vi "setIdx.vi"() -> ()   [LabVIEW 2016]
uses:
  OptStateEsti/OptStateEsti.lvclass
panel:
  out "dofIdx":i16[](array[numeric])
  out "DOF in Groups 2":T1
  out "zn3Idx 2":bool[](array[boolean])
  in  "DOF in Groups":T1
  in  "zn3Idx":bool[](array[boolean])
  in  "OptStateEsti in":refnum<class "OptStateEsti.lvclass">
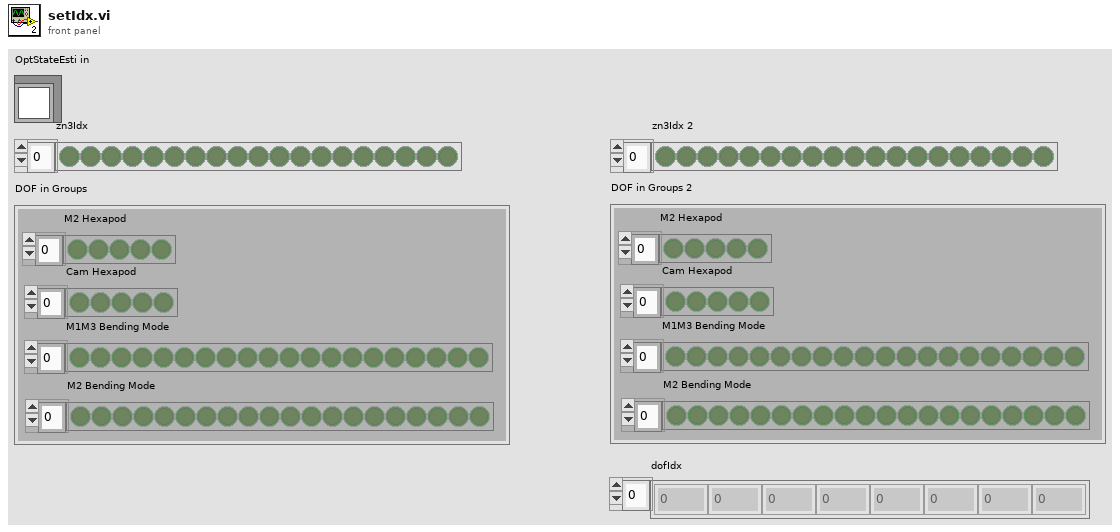
[diagram p1: front panel]
types:
  T1 = cluster{"M2 Hexapod":bool[], "Cam Hexapod ":bool[], "M1M3 Bending Mode":bool[], "M2 Bending Mode":bool[]}
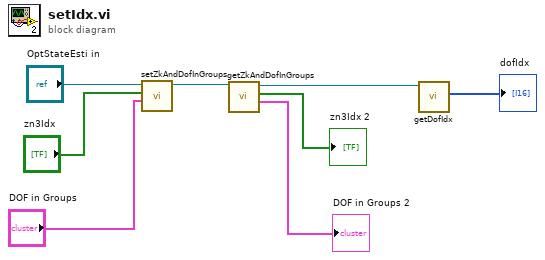
[diagram p0: block diagram]
diagram:
  n1 = call "setZkAndDofInGroups.vi"("DOF in Groups"="DOF in Groups", "zn3Idx"="zn3Idx", "OptStateEsti in"="OptStateEsti in") -> ("OptStateEsti out"=w8:refnum<class "OptStateEsti.lvclass">)  [unwired: 7 in, 1 out]
  n2 = call "getZkAndDofInGroups.vi"("OptStateEsti in"=w8) -> ("DOF in Groups"=→"DOF in Groups 2":T1, "zn3Idx"=→"zn3Idx 2":bool[], "OptStateEsti out"=w2:refnum<class "OptStateEsti.lvclass">)  [unwired: 7 in, 1 out]
  n3 = call "getDofIdx.vi"("OptStateEsti in"=w2) -> ("dofIdx"=→"dofIdx":i16[])  [unwired: 8 in, 2 out]
